vi "选择.vi"(6 "测试数据":dbl[][](array[numeric]), 7 "XY图":refnum<vi>, 8 "曲线设置":T1={"X轴数据选择"=enum."设置电压", "Y轴组"=[]}, 9 "数值":u32, 10 "错误输入（无错误）":errorcluster) -> (2 "错误输出":errorcluster)   [LabVIEW 2021]
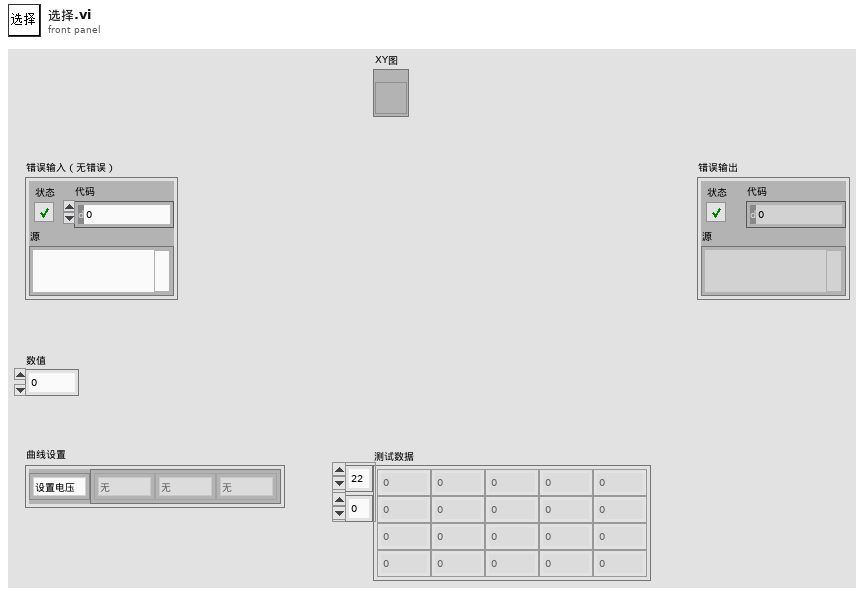
[diagram p1: front panel]
types:
  T1 = typedef "曲线设置.ctl" = cluster{"X轴数据选择":enum16{"时间", "设置电压", "读取电流", "读取电压"}, "Y轴组":enum16{"时间", "设置电压", "读取电流", "读取电压", "无"}[]}
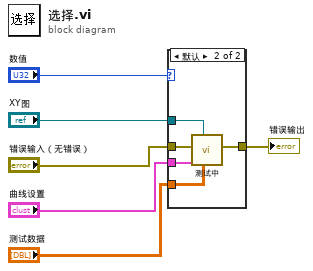
[diagram p0: block diagram]
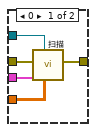
[diagram p2: hidden frame]
diagram:
  n1 = case shown="默认" "数值" {
    tunnel: "曲线设置" -> [w10 w16]
    tunnel: "测试数据" -> [w11 w12]
    tunnel: "XY图" -> [w8 w13]
    tunnel: "错误输入（无错误）" -> [w9 w15]
    tunnel: [w7 w14] -> w2
    frame 0 {
      n2 = call "扫描.vi"("测试数据"=w11, "XY图"=w8, "曲线设置"=w10, "错误输入（无错误）"=w9) -> ("错误输出"=w7:errorcluster)  [unwired: 7 in]
    }
    frame Default {
      n3 = call "测试中.vi"("测试数据"=w12, "XY图"=w13, "曲线设置"=w16, "错误输入（无错误）"=w15) -> ("错误输出"=w14:errorcluster)  [unwired: 7 in]
    }
  }
  "错误输出" <- w2
